vi "Sequence.BuildMain.vi"(6 "Iterations":u32, 8 "error in (no error)":errorcluster, 9 "Sequence Channels":T1, 10 "Steps":T3[](array[typedef]), 11 "Sequence":refnum<k24>) -> (0 "error out":errorcluster, 3 "Sequence out":refnum<k24>)   [LabVIEW 2013, in "Simple Sequence Tools - Editor.lvlib"]
uses:
  Simple Sequence Tools - Editor.lvlib
  NationalInstruments.VeriStand.RealTimeSequenceDefinitionApi
  Types/Compiled.StepProperties.ctl
  Types/Compiled.IOStateProperties.ctl
  Types/Compiled.StepElementProperties.ctl
  Shared/Types/Channel.Properties.ctl
  Shared/Types/Step.Types.ctl
  Types/Compiled.StepCondition.ctl
  Types/Conditions.OperationTypes.ctl
  Types/Compiled.SequenceChannels.ctl
  Shared/Simple Sequence Tools - Shared.lvlib
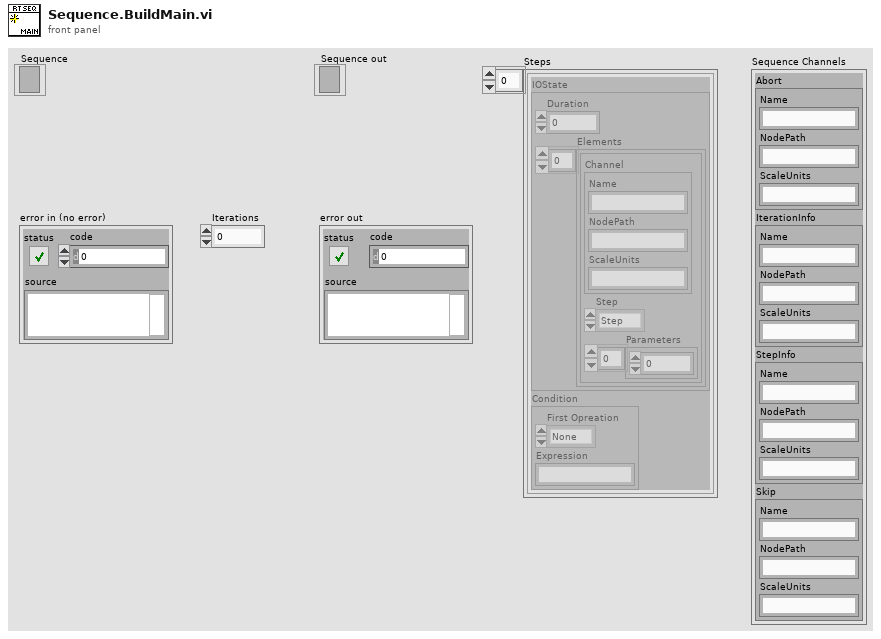
[diagram p1: front panel]
types:
  T1 = typedef "Simple Sequence Tools - Editor.lvlib/Compiled.SequenceChannels.ctl" = cluster{"Abort":T2, "IterationInfo":T2, "StepInfo":T2, "Skip":T2}
  T2 = typedef "Simple Sequence Tools - Shared.lvlib/Channel.Properties.ctl" = cluster{"Name":string, "NodePath":string, "ScaleUnits":string}
  T3 = typedef "Simple Sequence Tools - Editor.lvlib/Compiled.StepProperties.ctl" = cluster{"IOState":T4, "Condition":T7}
  T4 = typedef "Simple Sequence Tools - Editor.lvlib/Compiled.IOStateProperties.ctl" = cluster{"Duration":dbl, "Elements":T5[]}
  T5 = typedef "Simple Sequence Tools - Editor.lvlib/Compiled.StepElementProperties.ctl" = cluster{"Channel":T2, "Step":T6, "Parameters":dbl[]}
  T6 = typedef "Simple Sequence Tools - Shared.lvlib/Step.Types.ctl" = enum8{"Step", "iStep", "Ramp", "Unchanged", "Unknown", "Sine", "LogSine", "LinearSine", "ForcedRamp"}
  T7 = typedef "Simple Sequence Tools - Editor.lvlib/Compiled.StepCondition.ctl" = cluster{"First Opreation":T8, "Expression":string}
  T8 = typedef "Simple Sequence Tools - Editor.lvlib/Conditions.OperationTypes.ctl" = enum8{"None", "&&", "||"}
  T9 = typedef "Simple Sequence Tools - Editor.lvlib/Sequence.MainSeqRefs.ctl" = cluster{"Task.Main":refnum<k24>, "For.Main":refnum<k24>, "While.Main":refnum<k24>, "SelectCases.Main":refnum<k24>, "Switch.Main":refnum<k24>}
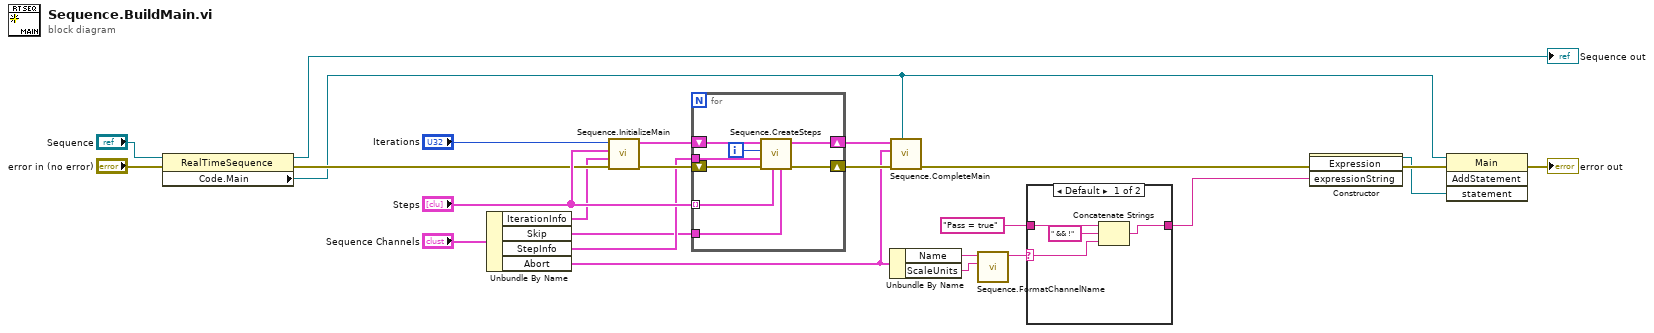
[diagram p0: block diagram]
diagram:
  n1 = property class="RealTimeSequence"(reference="Sequence", error in="error in (no error)") -> (reference out=→"Sequence out":refnum<k24>, error out=w19:errorcluster, "Code.Main"=w7:refnum<k24>)
  n2 = Unbundle By Name("Sequence Channels") -> ("IterationInfo"=w16:T2, "Skip"=w12:T2, "StepInfo"=w14:T2, "Abort"=w5:T2)
  n3 = call "Sequence.InitializeMain.vi"("error in (no error)"=w19, "IterationInfo"=w16, "Steps"="Steps", "Iterations"="Iterations") -> ("error out"=w22:errorcluster, "Refs"=w15:T9)  [unwired: 6 in]
  n4 = for {
    tunnel: "Steps" -> [w27] mode=indexing
    shift-right: [w33] -> w23
    shift-left: w22 -> [w30]
    tunnel: w14 -> [w31]
    shift-right: [w28] -> w13
    shift-left: w15 -> [w29]
    tunnel: w12 -> [w26]
    i -> [w32]
    n5 = call "Sequence.CreateSteps.vi"("Skip"=w26, "Step"=w27, "error in (no error)"=w30, "StepInfo"=w31, "Iteration"=w32, "Refs"=w29) -> ("error out"=w33:errorcluster, "Refs out"=w28:T9)  [unwired: 4 in]
  }
  n6 = Unbundle By Name(w5) -> ("Name"=w4:string, "ScaleUnits"=w3:string)
  n7 = call "Sequence.CompleteMain.vi"("Code.Main"=w7, "error in (no error)"=w23, "Abort"=w5, "Refs"=w13) -> ("error out"=w10:errorcluster)  [unwired: 7 in]
  n8 = call "Sequence.FormatChannelName.vi"("ScaleUnits"=w3, "Name"=w4) -> ("ChannelName"=w2:string)  [unwired: 9 in]
  n9 = case shown="Default" w2 {
    selector: w2 -> [w35 _]
    tunnel: [w34 w38] -> w6
    tunnel: "Pass = true" ("expressionString") -> [w37 w38]
    frame Default {
      n10 = Concatenate Strings(w37, " && !" ("string"), w35) -> (w34:string)
    }
    frame "\u0000" {
    }
  }
  n11 = constructor class="Expression"(error in=w10, "expressionString"=w6) -> (reference out=w8:refnum<k24>, error out=w9:errorcluster)  [unwired: 2 in, 2 out]
  n12 = invoke class="Main" method="AddStatement"(reference=w7, error in=w9, "statement"=w8) -> (error out=→"error out":errorcluster)  [unwired: 1 in, 3 out]
